vi "Create Asset JSON.vi"(4 "hardwareVersion":string, 5 "firmwareVersion":string, 6 "vendorNumber":i64, 7 "vendorName":string, 8 "modelNumber":i64, 9 "modelName":string, 10 "serialNumber":string, 11 "pluginName":string) -> (2 "JSON":string, 3 "File created?":bool)   [LabVIEW 2023, in "Utilities.lvlib"]
uses:
  Utilities.lvlib
  <vilib>/JDP Science/JSONtext/support/Format JSON Object.vi
  <vilib>/JDP Science/JSONtext/JSONtext.lvlib
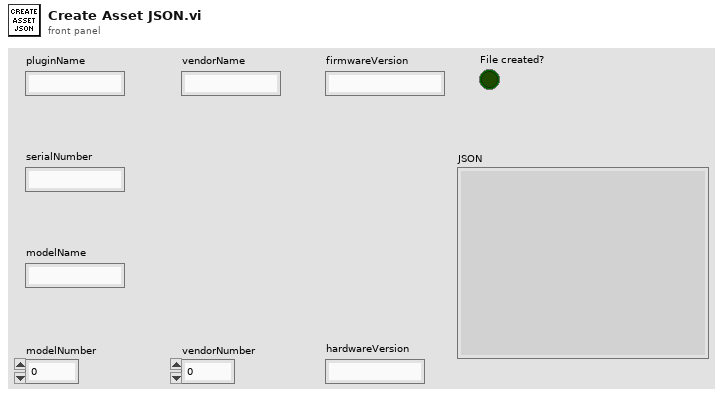
[diagram p1: front panel]
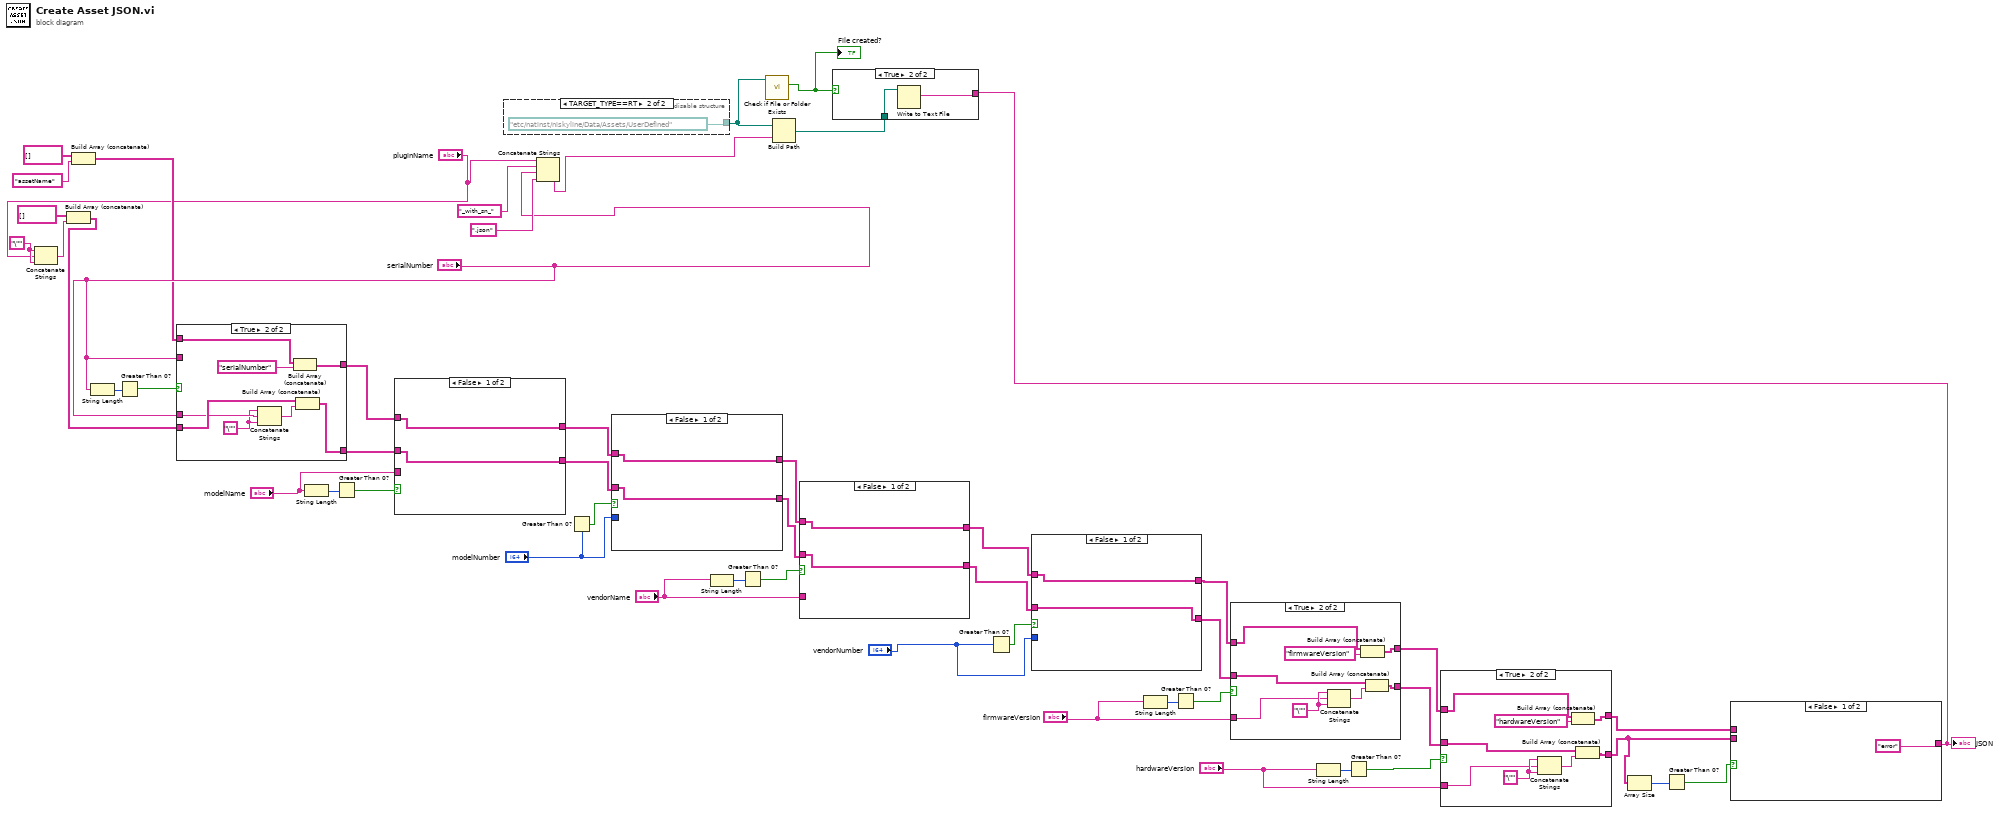
[diagram p0: block diagram]
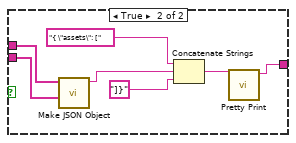
[diagram p3: hidden frame]
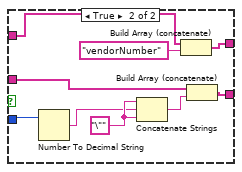
[diagram p6: hidden frame]
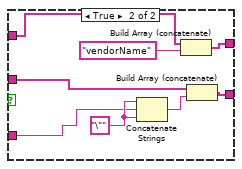
[diagram p7: hidden frame]
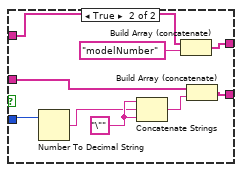
[diagram p8: hidden frame]
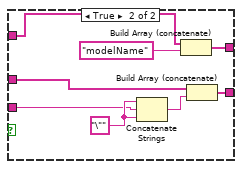
[diagram p9: hidden frame]
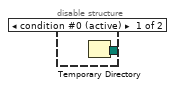
[diagram p11: hidden frame]
diagram:
  w8 = "\"" ("string")
  n1 = Concatenate Strings(w8, "pluginName", w8) -> (w7:string)
  n2 = Build Array (concatenate)(string[] [] ("array"), w7) -> (w5:string[])
  n3 = Build Array (concatenate)(string[] [] ("array"), "assetName" ("element")) -> (w4:string[])
  n4 = String Length(string="serialNumber") -> (length=w47:i32)
  n5 = Greater Than 0?(x=w47) -> (x > 0?=w46:bool)
  n6 = case shown="True" w46 {
    tunnel: "serialNumber" -> [_ _]
    tunnel: w4 -> [w52 w60]
    tunnel: [w52 w58] -> w45
    tunnel: w5 -> [w51 w57]
    tunnel: "serialNumber" -> [_ w55]
    tunnel: [w51 w53] -> w43
    frame False {
    }
    frame True {
      w54 = "\"" ("string")
      n7 = Concatenate Strings(w54, w55, w54) -> (w56:string)
      n8 = Build Array (concatenate)(w60, "serialNumber") -> (w58:string[])
      n9 = Build Array (concatenate)(w57, w56) -> (w53:string[])
    }
  }
  n10 = String Length(string="modelName") -> (length=w42:i32)
  n11 = Greater Than 0?(x=w42) -> (x > 0?=w40:bool)
  n12 = case shown="False" w40 {
    tunnel: w45 -> [w62 w69]
    tunnel: w43 -> [w61 w66]
    tunnel: "modelName" -> [_ w65]
    tunnel: [w62 w63] -> w39
    tunnel: [w61 w64] -> w38
    frame False {
    }
    frame True {
      w67 = "\"" ("string")
      n13 = Concatenate Strings(w67, w65, w67) -> (w68:string)
      n14 = Build Array (concatenate)(w69, "modelName") -> (w63:string[])
      n15 = Build Array (concatenate)(w66, w68) -> (w64:string[])
    }
  }
  n16 = disable-structure shown="TARGET_TYPE==RT" {
    disable-tunnel: [w71 path "/etc/natinst/niskyline/Data/Assets/UserDefined" ("path")] -> w12
    frame condition #0 (active) {
      n17 = Temporary Directory() -> (w71:path)
    }
    frame condition #1 {
    }
  }
  n18 = Concatenate Strings("pluginName", "_with_sn_" ("name or relative path"), "serialNumber", ".json" ("string")) -> (w48:string)
  n19 = Greater Than 0?(x="modelNumber") -> (x > 0?=w37:bool)
  n20 = case shown="False" w37 {
    tunnel: w39 -> [w74 w82]
    tunnel: w38 -> [w73 w79]
    tunnel: "modelNumber" -> [_ w77]
    tunnel: [w74 w76] -> w32
    tunnel: [w73 w75] -> w31
    frame False {
    }
    frame True {
      w80 = "\"" ("string")
      n21 = Number To Decimal String(number=w77) -> (decimal integer string=w78:string)  [unwired: 1 in]
      n22 = Concatenate Strings(w80, w78, w80) -> (w81:string)
      n23 = Build Array (concatenate)(w82, "modelNumber") -> (w76:string[])
      n24 = Build Array (concatenate)(w79, w81) -> (w75:string[])
    }
  }
  n25 = String Length(string="vendorName") -> (length=w35:i32)
  n26 = Greater Than 0?(x=w35) -> (x > 0?=w33:bool)
  n27 = call <vilib>:"Check if File or Folder Exists.vi"("path"=w12) -> ("file or folder exists?"=w9:bool)  [unwired: 8 in, 2 out]
  "File created?" <- w9
  n28 = Build Path(base path=w12, name or relative path=w48) -> (appended path=w10:path)
  n29 = case shown="False" w33 {
    tunnel: w32 -> [w85 w92]
    tunnel: w31 -> [w84 w89]
    tunnel: [w85 w88] -> w29
    tunnel: [w84 w87] -> w28
    tunnel: "vendorName" -> [_ w86]
    frame False {
    }
    frame True {
      w90 = "\"" ("string")
      n30 = Concatenate Strings(w90, w86, w90) -> (w91:string)
      n31 = Build Array (concatenate)(w92, "vendorName") -> (w88:string[])
      n32 = Build Array (concatenate)(w89, w91) -> (w87:string[])
    }
  }
  n33 = Greater Than 0?(x="vendorNumber") -> (x > 0?=w30:bool)
  n34 = case shown="False" w30 {
    tunnel: w29 -> [w95 w103]
    tunnel: w28 -> [w94 w100]
    tunnel: "vendorNumber" -> [_ w98]
    tunnel: [w95 w97] -> w26
    tunnel: [w94 w96] -> w25
    frame False {
    }
    frame True {
      w101 = "\"" ("string")
      n35 = Number To Decimal String(number=w98) -> (decimal integer string=w99:string)  [unwired: 1 in]
      n36 = Concatenate Strings(w101, w99, w101) -> (w102:string)
      n37 = Build Array (concatenate)(w103, "vendorNumber") -> (w97:string[])
      n38 = Build Array (concatenate)(w100, w102) -> (w96:string[])
    }
  }
  n39 = String Length(string="firmwareVersion") -> (length=w24:i32)
  n40 = Greater Than 0?(x=w24) -> (x > 0?=w23:bool)
  n41 = case shown="True" w23 {
    tunnel: w26 -> [w106 w113]
    tunnel: w25 -> [w105 w110]
    tunnel: [w106 w109] -> w17
    tunnel: [w105 w108] -> w18
    tunnel: "firmwareVersion" -> [_ w107]
    frame False {
    }
    frame True {
      w111 = "\"" ("string")
      n42 = Concatenate Strings(w111, w107, w111) -> (w112:string)
      n43 = Build Array (concatenate)(w113, "firmwareVersion") -> (w109:string[])
      n44 = Build Array (concatenate)(w110, w112) -> (w108:string[])
    }
  }
  n45 = String Length(string="hardwareVersion") -> (length=w21:i32)
  n46 = Greater Than 0?(x=w21) -> (x > 0?=w20:bool)
  n47 = case shown="True" w20 {
    tunnel: w17 -> [w116 w123]
    tunnel: w18 -> [w115 w120]
    tunnel: [w116 w119] -> w16
    tunnel: [w115 w118] -> w15
    tunnel: "hardwareVersion" -> [_ w117]
    frame False {
    }
    frame True {
      w121 = "\"" ("string")
      n48 = Concatenate Strings(w121, w117, w121) -> (w122:string)
      n49 = Build Array (concatenate)(w123, "hardwareVersion") -> (w119:string[])
      n50 = Build Array (concatenate)(w120, w122) -> (w118:string[])
    }
  }
  n51 = Array Size(array=w15) -> (size(s)=w14:i32)
  n52 = Greater Than 0?(x=w14) -> (x > 0?=w13:bool)
  n53 = case shown="False" w13 {
    tunnel: w15 -> [_ w130]
    tunnel: w16 -> [_ w129]
    tunnel: ["error" ("<JSON>") w126] -> w11
    frame False {
    }
    frame True {
      n54 = call <vilib>:"Make JSON Object.vi"("JSON Items"=w130, "Item Names"=w129) -> ("<JSON>"=w128:string)  [unwired: 8 in, 1 out]
      n55 = Concatenate Strings("{ \"assets\": [" ("string"), w128, "]}" ("string")) -> (w127:string)
      n56 = call <vilib>:"Pretty Print.vi"("JSON"=w127) -> ("<JSON>"=w126:string)  [unwired: 8 in, 2 out]
    }
  }
  "JSON" <- w11
  n57 = case shown="True" w9 {
    tunnel: w11 -> [_ w134]
    tunnel: w10 -> [_ w133]
    frame False {
    }
    frame True {
      n58 = Write to Text File(file (use dialog)=w133, text=w134) -> ()  [unwired: 2 in, 3 out]
    }
  }
